vi "BIN-date2daynum.vi"(2 "Time":timestamp) -> (7 "DayNum":u64)   [LabVIEW 2020]
doc: "Convert date to YYYYMMDD numerical value"
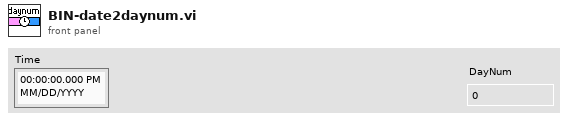
[diagram p1: front panel]
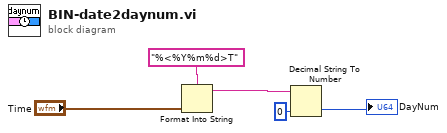
[diagram p0: block diagram]
diagram:
  n1 = Format Into String(format string="%<%Y%m%d>T", "Time") -> (resulting string=w2:string)  [unwired: 2 in, 1 out]
  n2 = Decimal String To Number(string=w2, default (0L)=u64 0 ("default (0 I32)")) -> (number=→"DayNum":u64)  [unwired: 1 in, 1 out]
